vi "TDK关闭.vi"(8 "error in (no error)":errorcluster, 11 "VISA resource name":refnum<visa-resource-name>) -> (0 "error out":errorcluster)   [LabVIEW 2021]
uses:
  <instrlib>/TDK-Lambda G Series/TDK-Lambda G Series.lvlib
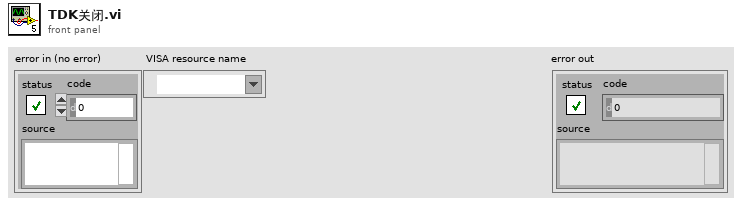
[diagram p1: front panel]
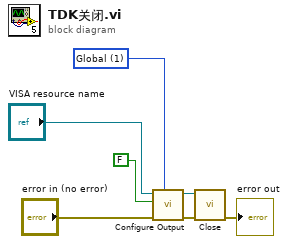
[diagram p0: block diagram]
diagram:
  w4 = u16 1 items=["Single", "Global"] ("Globalize (0: Single)")
  n1 = call <instrlib>:"Configure Output.vi"("Globalize (0: Single)"=w4, "error in (no error)"="error in (no error)", "Enable Output (False)"=FALSE ("Enable Output (True)"), "VISA resource name"="VISA resource name") -> ("error out"=w5:errorcluster, "VISA resource name out"=w6:refnum<visa-resource-name>)  [unwired: 6 in]
  n2 = call <instrlib>:"Close.vi"("error in (no error)"=w5, "VISA resource name"=w6) -> ("error out"=→"error out":errorcluster)  [unwired: 9 in]
